vi "Create New Logger.vi"(6 "Display Format":T1, 7 "Logger type":refnum<class "Logger.lvclass">, 8 "error in (no error)":errorcluster, 10 "Handlers":refnum<class "Handler.lvclass">[](array[class]), 11 "Name":string) -> (0 "error out":errorcluster, 3 "Logger out":refnum<class "Logger.lvclass">)   [LabVIEW 2017, in "Error Log.lvlib" / "Logger.lvclass"]
uses:
  Logger.lvclass
  Handler/Handler.lvclass
  Type Defs/Display Format.ctl
  Logger.lvclass/Logger.ctl
  Error Log.lvlib
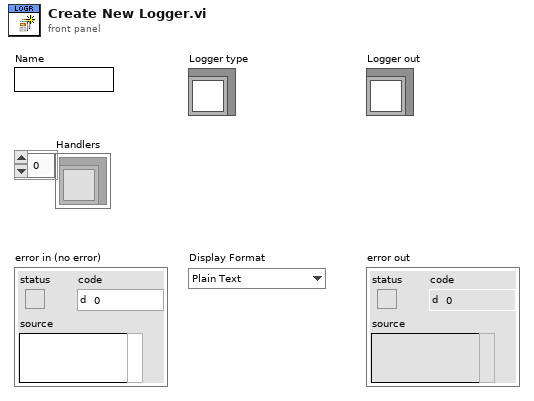
[diagram p1: front panel]
types:
  T1 = typedef "Error Log.lvlib/Display Format.ctl" = enum16{"Plain Text", "INI", "XML", "JSON"}
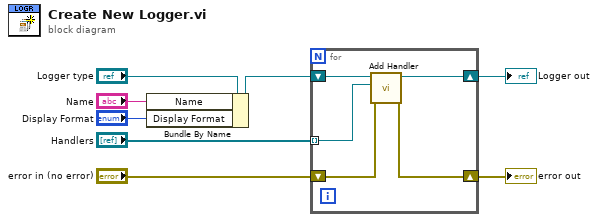
[diagram p0: block diagram]
diagram:
  n1 = Bundle By Name(cluster="Logger type", "Name"="Name", "Display Format"="Display Format") -> (w6:refnum<class "Logger.lvclass">)
  n2 = for {
    shift-right: [w12] -> w5
    shift-left: w6 -> [w13]
    shift-right: [w10] -> w3
    shift-left: "error in (no error)" -> [w11]
    tunnel: "Handlers" -> [w9] mode=indexing
    n3 = call "Add Handler.vi"("error in (no error)"=w11, "Handler"=w9, "Logger in"=w13) -> ("error out"=w10:errorcluster, "Logger out"=w12:refnum<class "Logger.lvclass">)  [unwired: 7 in]
  }
  "error out" <- w3
  "Logger out" <- w5
